vi "CreateValidFilePath_TU.vi"() -> ()   [LabVIEW 2025]
panel:
  out "path":path
  in  "folder  name":string
  in  "file name (no extension)":string
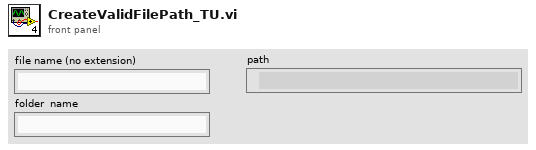
[diagram p1: front panel]
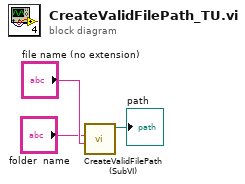
[diagram p0: block diagram]
diagram:
  n1 = call "CreateValidFilePath (SubVI).vi"("file name (no extension)"="file name (no extension)", "folder  name"="folder  name") -> ("path"=→"path":path)  [unwired: 9 in]
